vi "Run Beep.vi"(8 "error in (no error)":errorcluster, 10 "Beep Time [ms]":dbl=350.0, 11 "VISA resource name":refnum<visa-resource-name>) -> (0 "error out":errorcluster, 1 "Command Currently Unavailable":bool, 2 "Beep Done":bool, 3 "VISA resource name out":refnum<visa-resource-name>)   [LabVIEW 2017, in "RadWag balances and scales.lvlib"]
doc: "Runs internal beeper on seted time."
uses:
  <instrlib>/Radwag Balances and Scales/Public/RadWag balances and scales.lvlib
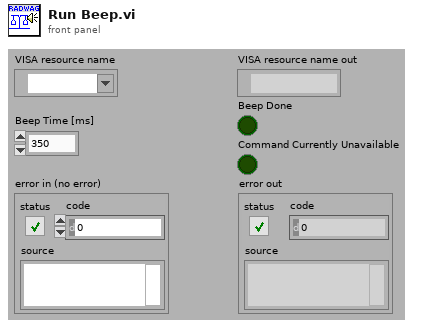
[diagram p1: front panel]
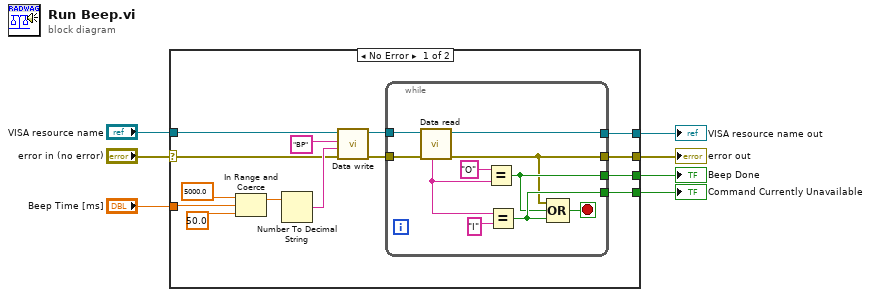
[diagram p0: block diagram]
diagram:
  n1 = case shown="No Error" "error in (no error)" {
    selector: "error in (no error)" -> [w8 w32]
    tunnel: "VISA resource name" -> [w14 w33]
    tunnel: "Beep Time [ms]" -> [w13 _]
    tunnel: [w12 w33] -> w4
    tunnel: [w11 _] -> w2
    tunnel: [w10 _] -> w1
    tunnel: [w9 w32] -> w3
    frame No Error {
      n2 = In Range and Coerce(upper limit=5000.0, x=w13, lower limit=50.0) -> (coerced(x)=w18:dbl)  [unwired: 1 out]
      n3 = Number To Decimal String(number=w18) -> (decimal integer string=w17:string)  [unwired: 1 in]
      n4 = call <instrlib>:"Data write.vi"("error in (no error)"=w8, "Parameter"=w17, "ID"="BP", "VISA resource name"=w14) -> ("error out"=w20:errorcluster, "VISA resource name out"=w21:refnum<visa-resource-name>)  [unwired: 6 in]
      n5 = while {
        tunnel: w21 -> [w31]
        tunnel: w20 -> [w30]
        tunnel: [w22] -> w12
        tunnel: [w23] -> w9
        tunnel: [w25] -> w10
        tunnel: [w24] -> w11
        stop <- w26 stop-if-true
        n6 = call <instrlib>:"Data read.vi"("error in (no error)"=w30, "VISA resource name"=w31) -> ("error out"=w23:errorcluster, "VISA resource name out"=w22:refnum<visa-resource-name>, "Status"=w29:string)  [unwired: 3 in, 4 out]
        n7 = Equal?(x="O", y=w29) -> (x = y?=w24:bool)
        n8 = Equal?(x=w29, y="I") -> (x = y?=w25:bool)
        n9 = Compound Arithmetic op=OR(w23, w24, w25) -> (w26:bool)
      }
    }
    frame Error {
    }
  }
  "VISA resource name out" <- w4
  "error out" <- w3
  "Beep Done" <- w2
  "Command Currently Unavailable" <- w1
